vi "StopData.vi"(8 "error in (no error)":errorcluster, 11 "RoomAlertIn":refnum<class "RoomAlert.lvclass">) -> (0 "error out":errorcluster, 3 "RoomAlertOut":refnum<class "RoomAlert.lvclass">)   [LabVIEW 2018, in "SensorPlugins.lvlib" / "RoomAlert.lvclass"]
doc: "Stops the RoomAlert measurements."
uses:
  RoomAlert.lvclass
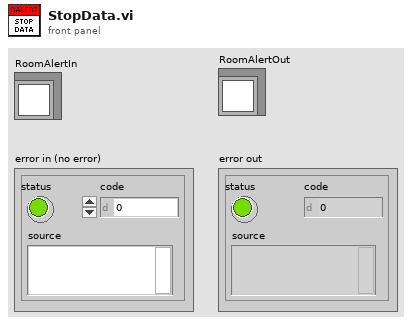
[diagram p1: front panel]
types:
  T1 = typedef "SensorPlugins.lvlib/RoomAlert.lvclass/MeasurementControls.ctl" = cluster{"Measurement RefreshTime (ms)":u32, "Measurement Name":string, "Timeout(ms)":i32, "Amber Warning Light Configuration":cluster{"Warning Temperture (Degrees C)":dbl, "Temperature Delta (Degrees C/Minute)":dbl, "Time Window (Minutes)":dbl}}
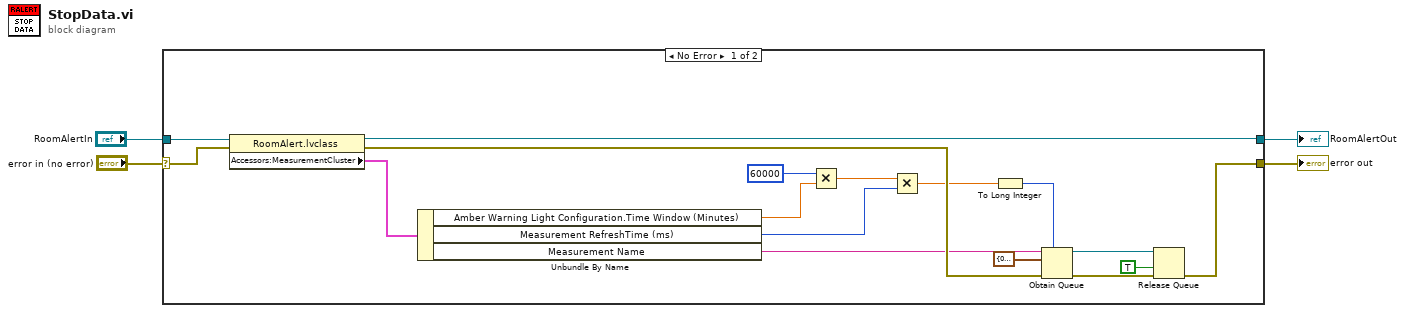
[diagram p0: block diagram]
diagram:
  n1 = case shown="No Error" "error in (no error)" {
    selector: "error in (no error)" -> [w11 w22]
    tunnel: "RoomAlertIn" -> [w12 w23]
    tunnel: [w20 w22] -> w2
    tunnel: [w8 w23] -> w1
    frame No Error {
      n2 = property class="RoomAlert.lvclass"(reference=w12, error in=w11) -> (reference out=w8:refnum<class "RoomAlert.lvclass">, error out=w19:errorcluster, "Accessors:MeasurementCluster"=w17:T1)
      n3 = Unbundle By Name(w17) -> ("Amber Warning Light Configuration.Time Window (Minutes)"=w14:dbl, "Measurement RefreshTime (ms)"=w16:u32, "Measurement Name"=w18:string)
      n4 = Multiply(x=60000 ("y"), y=w14) -> (x*y=w15:dbl)
      n5 = Multiply(x=w15, y=w16) -> (x*y=w7:dbl)
      n6 = To Long Integer(number=w7) -> (32bit integer=w6:i32)
      n7 = Obtain Queue(max queue size (-1, unlimited)=w6, name (unnamed)=w18, element data type=cluster{"Temp1":dbl, "Temp2":dbl} {"Temp1"=0.0, "Temp2"=0.0} ("Cluster"), error in (no error)=w19) -> (queue out=w9:refnum<queue>, error out=w10:errorcluster)  [unwired: 1 in, 1 out]
      n8 = Release Queue(queue=w9, force destroy? (F)=TRUE, error in (no error)=w10) -> (error out=w20:errorcluster)  [unwired: 2 out]
    }
    frame Error {
    }
  }
  "RoomAlertOut" <- w1
  "error out" <- w2
